vi "Set Transfer Group Transfers.vi"(8 "error in (no error)":errorcluster, 10 "transfers":T1[](array[typedef]) {"channels"."string offset" format="%d bytes"}, 11 "transfer group in":T6={"name"="Group", "direction"=enum."Tx", "cycle timing"={"priority"=100, "decimation"=1, "offset"=0}, "thread index"=255, "settings"=[], "transfers"=[], "timeout behavior"=enum."Increment Late Count", "convert buffers"=FALSE} {"transfers"."channels"."string offset" format="%d bytes"}) -> (0 "error out":errorcluster, 3 "transfer group out":T6={"name"="Group", "direction"=enum."Tx", "cycle timing"={"priority"=100, "decimation"=1, "offset"=0}, "thread index"=255, "settings"=[], "transfers"=[], "timeout behavior"=enum."Increment Late Count", "convert buffers"=FALSE} {"transfers"."channels"."string offset" format="%d bytes"})   [LabVIEW 2017, in "DSF Core.lvlib" / "Configuration Session.lvclass"]
uses:
  Configuration Session.lvclass
  Typedefs/DSF Engine Transfer Group Configuration.ctl
  Typedefs/DSF Direction.ctl
  Typedefs/DSF Timing Info.ctl
  Typedefs/DSF Settings Info.ctl
  Typedefs/DSF Engine Transfer Configuration.ctl
  Typedefs/DSF Byte Order.ctl
  Typedefs/DSF Engine Channel Configuration.ctl
  Typedefs/DSF Data Type.ctl
  Typedefs/DSF Timeout Behavior.ctl
  DSF Core.lvlib
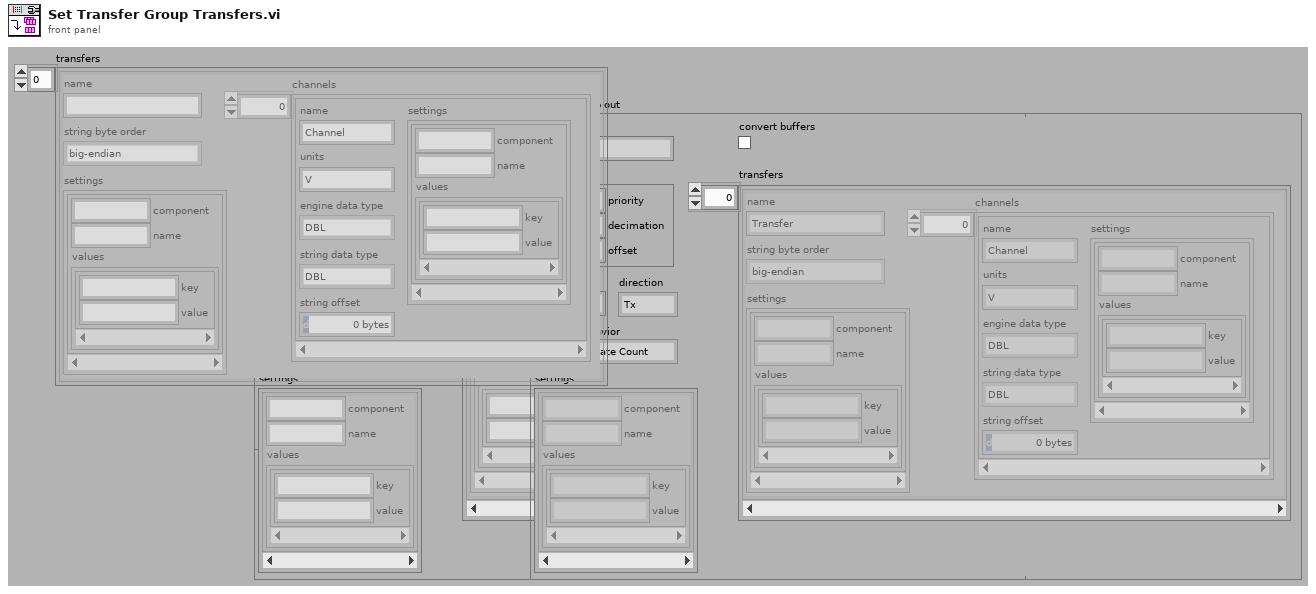
[diagram p1: front panel]
types:
  T1 = typedef "DSF Core.lvlib/DSF Engine Transfer Configuration.ctl" = cluster{"name":string, "string byte order":T2, "settings":T3, "channels":T4[]}
  T2 = typedef "DSF Core.lvlib/DSF Byte Order.ctl" = enum8{"big-endian", "little-endian"}
  T3 = typedef "DSF Core.lvlib/DSF Settings Info.ctl" = cluster{"component":string, "name":string, "values":cluster{"key":string, "value":string}[]}[]
  T4 = typedef "DSF Core.lvlib/DSF Engine Channel Configuration.ctl" = cluster{"string offset":u64, "name":string, "units":string, "engine data type":T5, "string data type":T5, "settings":T3}
  T5 = typedef "DSF Core.lvlib/DSF Data Type.ctl" = enum8{"Bool", "SGL", "DBL", "I8", "I16", "I32", "I64", "U8", "U16", "U32", "U64"}
  T6 = typedef "DSF Core.lvlib/DSF Engine Transfer Group Configuration.ctl" = cluster{"name":string, "direction":T7, "cycle timing":T8, "thread index":u8, "settings":T3, "transfers":T1[], "timeout behavior":T9, "convert buffers":bool}
  T7 = typedef "DSF Core.lvlib/DSF Direction.ctl" = enum8{"Tx", "Rx"}
  T8 = typedef "DSF Core.lvlib/DSF Timing Info.ctl" = cluster{"priority":u64, "decimation":u64, "offset":u64}
  T9 = typedef "DSF Core.lvlib/DSF Timeout Behavior.ctl" = enum8{"Increment Late Count", "Throw Error"}
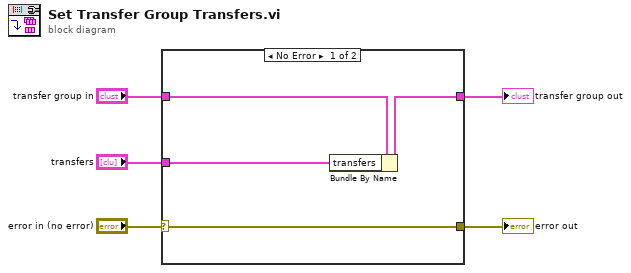
[diagram p0: block diagram]
diagram:
  n1 = case shown="No Error" "error in (no error)" {
    selector: "error in (no error)" -> [w7 w11]
    tunnel: [w7 w11] -> w5
    tunnel: [w8 w10] -> w2
    tunnel: "transfer group in" -> [w9 w10]
    tunnel: "transfers" -> [w6 _]
    frame No Error {
      n2 = Bundle By Name(cluster=w9, "transfers"=w6) -> (w8:T6)
    }
    frame Error {
    }
  }
  "error out" <- w5
  "transfer group out" <- w2
